vi "CH_LM DFM Copy File.vi"(0 "Meter Index":i32, 1 "Source Name (\"\")":string, 2 "Destination Name (\"\")":string, 5 "error in (no error)":errorcluster, 7 "Timeout / ms (3000)":i32=3000, 9 "Lock Timeout / ms (1000)":i32=1000) -> (11 "Lock timed out":bool, 14 "Meter Index":i32, 19 "error out":errorcluster)   [LabVIEW 2012, in "CH_LM.lvlib"]
doc: "This command will copy a source file to a destination. The source parameter will indicate a relative or absolute source path to an existing file. The destination parameter may indicate a relative or absolute path to a new non-existent destination file or an existing destination directory. The current working directory is assumed if the directory component of either source or destination path is omitted. A duplicate of the source file will be created with the destination file name in the specified directory if the destination parameter represents a file. A duplicate of the source file will be created with the same source file name in the specified directory if the destination parameter represents a directory. Copying a file requires that the \".csv\" file name extension be specified for source files and destination file names (not destination directories).\n\n<B>Attention:</B> An attempt to copy a file that does not exist will raise error 201. An attempt to copy a file to a destination file that already exists will raise error 202 or 203 depending if the destination is a directory or a file. An attempt to copy a file when the storage media is full will raise error -254. An attempt to copy a source file that is currently in use will raise error 101.\n\n<B>Note</B> that file copies may be lengthy operations. For this reason they are performed in the background. The result code returned by this command represents a \"good faith\" effort at predicting the results of the subsequent copy operation. If the background copy ultimately fails error -200 will be raised after the initial reply to this command has been returned. The system status word contains a bit to indicate that a host file copy is in progress. The host may check this bit to see if any copies are in progress."
uses:
  CH_LM.lvlib
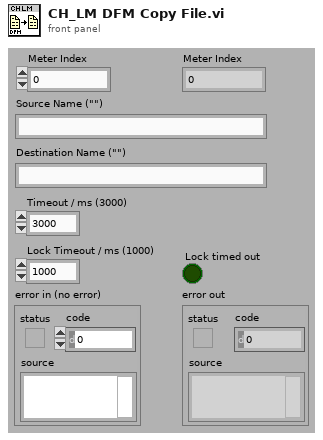
[diagram p1: front panel]
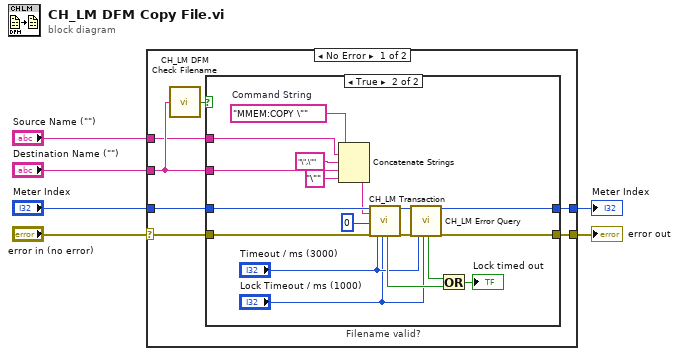
[diagram p0: block diagram]
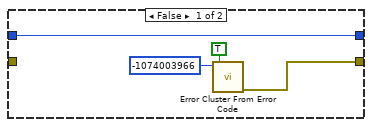
[diagram p2: hidden frame]
diagram:
  n1 = case shown="No Error" "error in (no error)" {
    selector: "error in (no error)" -> [w13 w37]
    tunnel: [w10 w37] -> w6
    tunnel: "Meter Index" -> [w12 w36]
    tunnel: [w11 w36] -> w3
    tunnel: "Destination Name (\"\")" -> [w8 _]
    tunnel: "Source Name (\"\")" -> [w7 _]
    frame No Error {
      n2 = call "CH_LM DFM Check Filename.vi"("Directory or File Name (\"\")"=w8) -> ("Valid"=w9:bool)
      n3 = case "Filename valid?" shown="True" w9 {
        tunnel: w13 -> [_ w35]
        tunnel: w12 -> [w14 w34]
        tunnel: [w14 w30] -> w11
        tunnel: [w15 w29] -> w10
        tunnel: w8 -> [_ w23]
        tunnel: w7 -> [_ w19]
        frame False {
          n4 = call <vilib>:"Error Cluster From Error Code.vi"("show call chain? (False)"=TRUE, "error code (0)"=-1074003966) -> ("error out"=w15:errorcluster)  [unwired: 1 in, 6 out]
        }
        frame True {
          w18 = "MMEM:COPY \""  # Command String
          n5 = Concatenate Strings(w18, w19, "\",\"" ("string"), w23, "\"" ("string")) -> (w22:string)
          n6 = call "CH_LM Transaction.vi"("Meter Index"=w34, "Command String"=w22, "NofStrings (-1:all)"=0 ("t"), "error in (no error)"=w35, "Timeout / ms (3000)"="Timeout / ms (3000)", "Lock Timeout / ms (1000)"="Lock Timeout / ms (1000)") -> ("Lock timed out"=w27:bool, "Meter Index"=w32:i32, "error out"=w31:errorcluster)  [unwired: 11 out]
          n7 = call "CH_LM Error Query.vi"("Meter Index"=w32, "error in (no error)"=w31, "Timeout / ms (3000)"="Timeout / ms (3000)", "Lock Timeout / ms (1000)"="Lock Timeout / ms (1000)") -> ("Lock timed out"=w28:bool, "Meter Index"=w30:i32, "error out"=w29:errorcluster)  [unwired: 13 out]
          n8 = Or(x=w28, y=w27) -> (x .or. y?=→"Lock timed out":bool)
        }
      }
    }
    frame Error {
    }
  }
  "error out" <- w6
  "Meter Index" <- w3
